vi "WebView2_ParsePostMessage.vi"(11 "WebMessageAsJson":string) -> (1 "ItemName":string, 2 "ItemVI":path, 3 "Action":string)   [LabVIEW 2020, in "WebView2-Viewer.lvlib"]
uses:
  WebView2-Viewer.lvlib
panel:
  out "value 4":T1
  out "value 2":T2
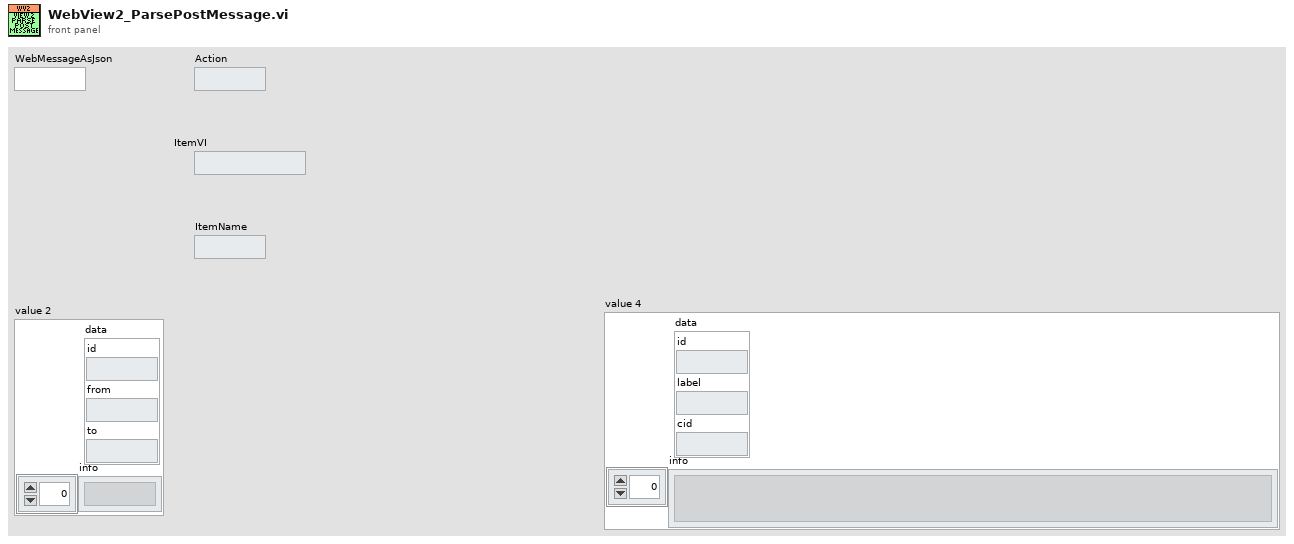
[diagram p1: front panel]
types:
  T1 = cluster{"data":cluster{"id":string, "label":string, "cid":string}, "info":string[]}
  T2 = cluster{"data":cluster{"id":string, "from":string, "to":string}, "info":string[]}
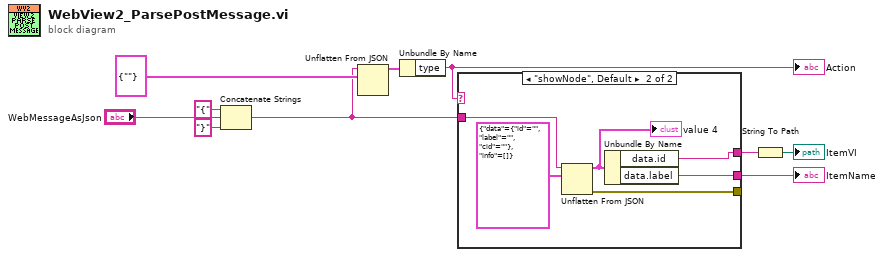
[diagram p0: block diagram]
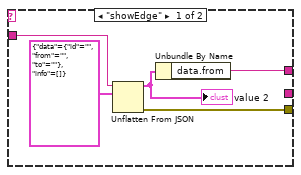
[diagram p2: hidden frame]
diagram:
  n1 = Concatenate Strings("{" ("string"), "WebMessageAsJson", "}" ("string")) -> (w3:string)
  n2 = Unflatten From JSON(JSON string=w3, type and defaults=cluster{"type":string} {"type"=""}) -> (value=w9:cluster{"type":string})  [unwired: 5 in, 1 out]
  n3 = Unbundle By Name(w9) -> ("type"=w8:string)
  "Action" <- w8
  n4 = case shown="\"showNode\", Default" w8 {
    tunnel: w3 -> [w14 w20]
    tunnel: [w13 w19] -> _
    tunnel: [w11 w17] -> w6
    tunnel: [_ w16] -> w5
    frame "showEdge" {
      n5 = Unflatten From JSON(JSON string=w14, type and defaults=T2 {"data"={"id"="", "from"="", "to"=""}, "info"=[]}) -> (value=w12:T2, error out=w13:errorcluster)  [unwired: 5 in]
      "value 2" <- w12
      n6 = Unbundle By Name(w12) -> ("data.from"=w11:string)
    }
    frame "showNode", Default {
      n7 = Unflatten From JSON(JSON string=w20, type and defaults=T1 {"data"={"id"="", "label"="", "cid"=""}, "info"=[]}) -> (value=w18:T1, error out=w19:errorcluster)  [unwired: 5 in]
      "value 4" <- w18
      n8 = Unbundle By Name(w18) -> ("data.id"=w17:string, "data.label"=w16:string)
    }
  }
  "ItemName" <- w5
  n9 = String To Path(string=w6) -> (path=→"ItemVI":path)
